vi "Finish.vi"   [LabVIEW 2016]
doc: "This VI is called just before exiting. It is expected to close I/O refnum, save collected data, etc."
uses:
  <vilib>/Rock Robotics/WPI/Utilities/WPI_GetSetVariantRefNum.vi
types:
  T1 = typedef "WPI_MotorControlDeviceRef.ctl" = cluster{"DeviceStatus":errorcluster, "Type":T2, "PWM":cluster{"PWM Channel":T3, "DeadBand":T4}, "CAN":cluster{"Device Number":u8, "SetOutput VI Ref":variant, "GetOutput VI Ref":variant, "Enable VI Ref":variant, "Disable VI Ref":variant, "Data":variant}, "Invert":bool}
  T2 = typedef "WPI_MotorControlType.ctl" = enum16{"PWM", "CAN"}
  T3 = typedef "FPGA_DIOPWMChannel.ctl" = enum8{"PWM 0", "PWM 1", "PWM 2", "PWM 3", "PWM 4", "PWM 5", "PWM 6", "PWM 7", "PWM 8", "PWM 9", "PWM MXP 0", "PWM MXP 1", "PWM MXP 2", "PWM MXP 3", "PWM MXP 4", "PWM MXP 5", "PWM MXP 6", "PWM MXP 7", "PWM MXP 8", "PWM MXP 9", "Invalid"}
  T4 = typedef "WPI_PWMDeadband.ctl" = cluster{"Name":string, "maxPositivePwm":i32, "minPositivePwm":i32, "centerPwm":i32, "maxNegativePwm":i32, "minNegativePwm":i32, "angularRange":u16}
  T5 = typedef "WPI_JoystickDevRef.ctl" = cluster{"Device":T6}
  T6 = typedef "WPI_JoystickDeviceEnum.ctl" = enum16{"USB 0", "USB 1", "USB 2", "USB 3", "USB 4", "USB 5"}
  T7 = typedef "WPI_SolenoidDevRef.ctl" = cluster{"DevStatus":errorcluster, "Pneumatics Control Module":u8, "Forward Solenoid Channel":T8, "Reverse Solenoid Channel":T8}
  T8 = typedef "WPI_SolenoidChannel.ctl" = enum8{"Solenoid 0", "Solenoid 1", "Solenoid 2", "Solenoid 3", "Solenoid 4", "Solenoid 5", "Solenoid 6", "Solenoid 7", "Invalid"}
  T9 = typedef "WPI_GyroDevRef.ctl" = cluster{"DevStatus":errorcluster, "Analog Channel":T10, "Offset":dbl, "Gain (VoltsPerDegree/Second)":dbl, "Gyro Type":enum16{"Analog", "XRS450"}, "Handle":i32, "SPI Bus":T11, "Device Found":bool, "Sample Rate":dbl, "Calibrate On Open":bool}
  T10 = typedef "FPGA_AIChannel.ctl" = enum8{"AI 0", "AI 1", "AI 2", "AI 3", "AI MXP 0", "AI MXP 1", "AI MXP 2", "AI MXP 3", "Invalid"}
  T11 = typedef "spi_bus.ctl" = enum16{"SPI On-Board, CS0", "SPI On-Board, CS1", "SPI On-Board, CS2", "SPI On-Board, CS3", "SPI MXP", "Invalid"}
  T12 = typedef "WPI_EncoderDevRef.ctl" = cluster{"DevStatus":errorcluster, "EncoderIndex":T13, "CounterIndex":T14, "DistancePerCount":dbl, "Decoding Type":T15}
  T13 = typedef "FPGA_EncoderIdx.ctl" = enum8{"Enc 0", "Enc 1", "Enc 2", "Enc 3", "Enc 4", "Enc 5", "Enc 6", "Enc 7", "Invalid"}
  T14 = typedef "FPGA_CounterCtrSystemIndex.ctl" = enum8{"Ctr 0", "Ctr 1", "Ctr 2", "Ctr 3", "Ctr 4", "Ctr 5", "Ctr 6", "Ctr 7", "Invalid"}
  T15 = typedef "WPI_EncoderType.ctl" = enum16{"1x", "2x", "4x"}
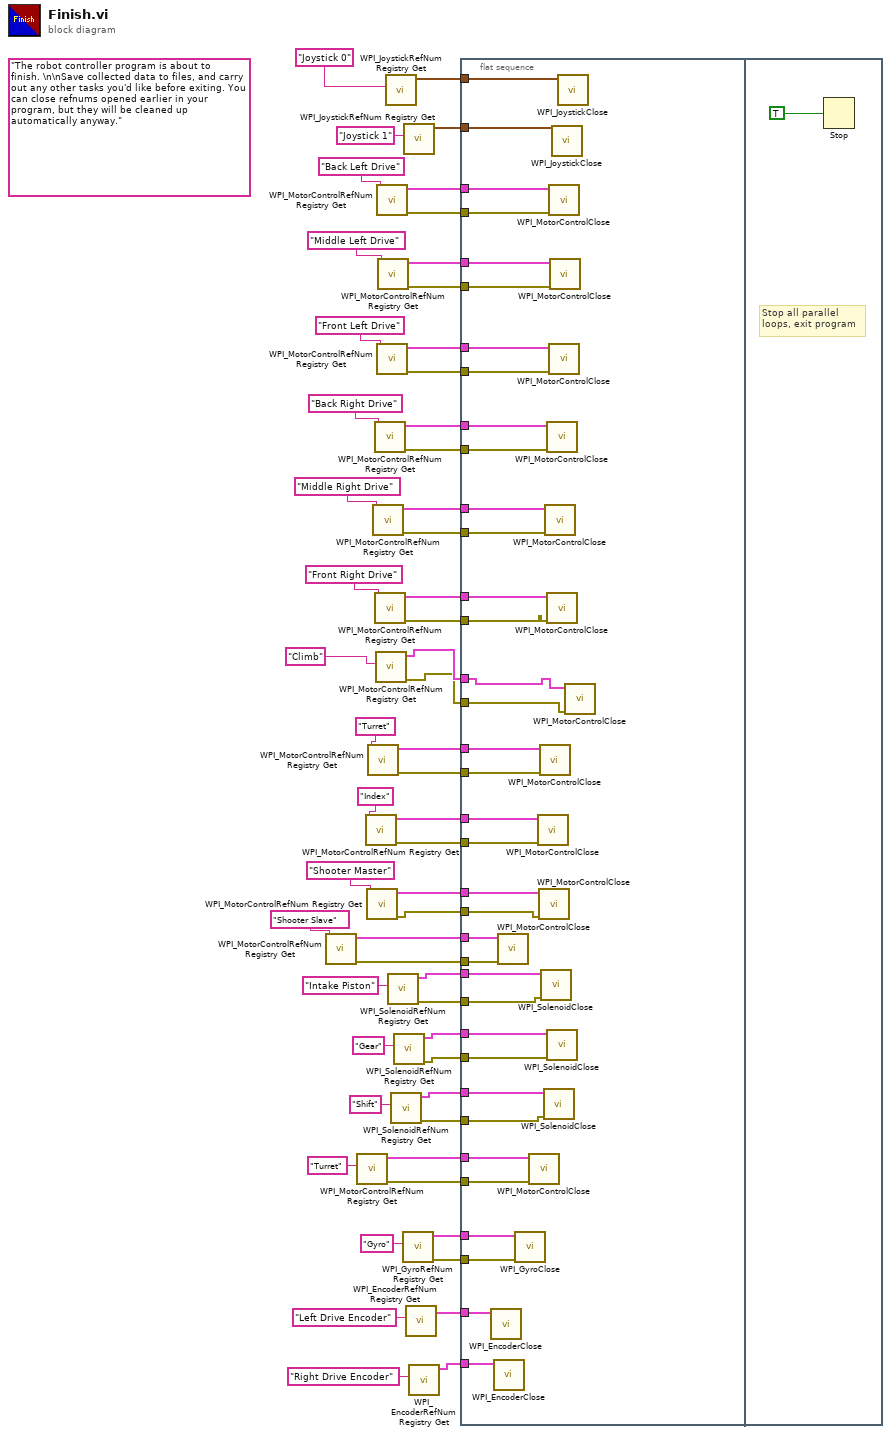
[diagram p0: block diagram]
diagram:
  (unwired) "The robot controller program is about to finish. \n\nSave collected data to files, and carry out any other tasks you'd like before exiting. You can close refnums opened earlier in your program, but they will be cleaned up automatically anyway."
  n1 = call <vilib>:"WPI_MotorControlRefNum Registry Get.vi"("refnum name"="Shooter Slave") -> ("error out"=w21:errorcluster, "MotorControlDevRef"=w31:T1)  [unwired: 9 in]
  n2 = call <vilib>:"WPI_MotorControlRefNum Registry Get.vi"("refnum name"="Turret") -> ("error out"=w16:errorcluster, "MotorControlDevRef"=w28:T1)  [unwired: 9 in]
  n3 = call <vilib>:"WPI_MotorControlRefNum Registry Get.vi"("refnum name"="Index") -> ("error out"=w23:errorcluster, "MotorControlDevRef"=w35:T1)  [unwired: 9 in]
  n4 = call <vilib>:"WPI_MotorControlRefNum Registry Get.vi"("refnum name"="Shooter Master") -> ("error out"=w20:errorcluster, "MotorControlDevRef"=w34:T1)  [unwired: 9 in]
  n5 = call <vilib>:"WPI_MotorControlRefNum Registry Get.vi"("refnum name"="Turret") -> ("error out"=w22:errorcluster, "MotorControlDevRef"=w38:T1)  [unwired: 9 in]
  n6 = call <vilib>:"WPI_MotorControlRefNum Registry Get.vi"("refnum name"="Middle Right Drive") -> ("error out"=w25:errorcluster, "MotorControlDevRef"=w41:T1)  [unwired: 9 in]
  n7 = call <vilib>:"WPI_MotorControlRefNum Registry Get.vi"("refnum name"="Back Right Drive") -> ("error out"=w24:errorcluster, "MotorControlDevRef"=w44:T1)  [unwired: 9 in]
  n8 = call <vilib>:"WPI_MotorControlRefNum Registry Get.vi"("refnum name"="Front Right Drive") -> ("error out"=w26:errorcluster, "MotorControlDevRef"=w40:T1)  [unwired: 9 in]
  n9 = call <vilib>:"WPI_MotorControlRefNum Registry Get.vi"("refnum name"="Climb") -> ("error out"=w10:errorcluster, "MotorControlDevRef"=w11:T1)  [unwired: 9 in]
  n10 = call <vilib>:"WPI_MotorControlRefNum Registry Get.vi"("refnum name"="Back Left Drive") -> ("error out"=w13:errorcluster, "MotorControlDevRef"=w54:T1)  [unwired: 9 in]
  n11 = call <vilib>:"WPI_MotorControlRefNum Registry Get.vi"("refnum name"="Front Left Drive") -> ("error out"=w15:errorcluster, "MotorControlDevRef"=w45:T1)  [unwired: 9 in]
  n12 = call <vilib>:"WPI_MotorControlRefNum Registry Get.vi"("refnum name"="Middle Left Drive") -> ("error out"=w14:errorcluster, "MotorControlDevRef"=w48:T1)  [unwired: 9 in]
  n13 = call <vilib>:"WPI_JoystickRefNum Registry Get.vi"("refnum name"="Joystick 0") -> ("JoystickDevRef"=w53:T5)  [unwired: 1 in, 9 out]
  n14 = call <vilib>:"WPI_SolenoidRefNum Registry Get.vi"("refnum name"="Intake Piston") -> ("error out"=w19:errorcluster, "SolenoidDevRef"=w51:T7)  [unwired: 9 in]
  n15 = call <vilib>:"WPI_SolenoidRefNum Registry Get.vi"("refnum name"="Shift") -> ("error out"=w17:errorcluster, "SolenoidDevRef"=w29:T7)  [unwired: 9 in]
  n16 = call <vilib>:"WPI_SolenoidRefNum Registry Get.vi"("refnum name"="Gear") -> ("error out"=w18:errorcluster, "SolenoidDevRef"=w50:T7)  [unwired: 9 in]
  n17 = call <vilib>:"WPI_GyroRefNum Registry Get.vi"("refnum name"="Gyro") -> ("error out"=w6:errorcluster, "GyroDevRef"=w7:T9)  [unwired: 9 in]
  n18 = call <vilib>:"WPI_JoystickRefNum Registry Get.vi"("refnum name"="Joystick 1") -> ("JoystickDevRef"=w8:T5)  [unwired: 9 in, 1 out]
  n19 = call <vilib>:"WPI_EncoderRefNum Registry Get.vi"("refnum name"="Left Drive Encoder") -> ("EncoderDevRef"=w2:T12)  [unwired: 9 in, 1 out]
  n20 = call <vilib>:"WPI_EncoderRefNum Registry Get.vi"("refnum name"="Right Drive Encoder") -> ("EncoderDevRef"=w1:T12)  [unwired: 9 in, 1 out]
  n21 = flat-sequence {
    tunnel: w54 -> [w89]
    tunnel: w53 -> [w92]
    tunnel: w51 -> [w91]
    tunnel: w50 -> [w90]
    tunnel: w48 -> [w88]
    tunnel: w45 -> [w87]
    tunnel: w44 -> [w86]
    tunnel: w41 -> [w85]
    tunnel: w40 -> [w84]
    tunnel: w11 -> [w63]
    tunnel: w38 -> [w83]
    tunnel: w35 -> [w82]
    tunnel: w34 -> [w81]
    tunnel: w31 -> [w80]
    tunnel: w29 -> [w79]
    tunnel: w28 -> [w78]
    tunnel: w10 -> [w62]
    tunnel: w26 -> [w77]
    tunnel: w25 -> [w76]
    tunnel: w24 -> [w75]
    tunnel: w23 -> [w74]
    tunnel: w22 -> [w73]
    tunnel: w21 -> [w72]
    tunnel: w20 -> [w71]
    tunnel: w19 -> [w70]
    tunnel: w18 -> [w69]
    tunnel: w17 -> [w68]
    tunnel: w16 -> [w67]
    tunnel: w15 -> [w66]
    tunnel: w14 -> [w65]
    tunnel: w13 -> [w64]
    tunnel: w8 -> [w61]
    tunnel: w7 -> [w60]
    tunnel: w6 -> [w59]
    tunnel: w2 -> [w58]
    tunnel: w1 -> [w57]
    frame #0 {
      n22 = call <vilib>:"WPI_EncoderClose.vi"("EncoderDevRef"=w58) -> ()  [unwired: 10 in, 1 out]
      n23 = call <vilib>:"WPI_EncoderClose.vi"("EncoderDevRef"=w57) -> ()  [unwired: 10 in, 1 out]
      n24 = call <vilib>:"WPI_MotorControlClose.vi"("error in"=w72, "MotorControlDevRef"=w80) -> ()  [unwired: 9 in, 1 out]
      n25 = call <vilib>:"WPI_GyroClose.vi"("error in"=w59, "GyroDevRef"=w60) -> ()  [unwired: 9 in, 1 out]
      n26 = call <vilib>:"WPI_MotorControlClose.vi"("error in"=w67, "MotorControlDevRef"=w78) -> ()  [unwired: 9 in, 1 out]
      n27 = call <vilib>:"WPI_MotorControlClose.vi"("error in"=w74, "MotorControlDevRef"=w82) -> ()  [unwired: 9 in, 1 out]
      n28 = call <vilib>:"WPI_MotorControlClose.vi"("error in"=w71, "MotorControlDevRef"=w81) -> ()  [unwired: 9 in, 1 out]
      n29 = call <vilib>:"WPI_MotorControlClose.vi"("error in"=w73, "MotorControlDevRef"=w83) -> ()  [unwired: 9 in, 1 out]
      n30 = call <vilib>:"WPI_SolenoidClose.vi"("error in (no error)"=w70, "SolenoidDevRef"=w91) -> ()  [unwired: 9 in, 1 out]
      n31 = call <vilib>:"WPI_SolenoidClose.vi"("error in (no error)"=w68, "SolenoidDevRef"=w79) -> ()  [unwired: 9 in, 1 out]
      n32 = call <vilib>:"WPI_MotorControlClose.vi"("error in"=w76, "MotorControlDevRef"=w85) -> ()  [unwired: 9 in, 1 out]
      n33 = call <vilib>:"WPI_MotorControlClose.vi"("error in"=w75, "MotorControlDevRef"=w86) -> ()  [unwired: 9 in, 1 out]
      n34 = call <vilib>:"WPI_MotorControlClose.vi"("error in"=w77, "MotorControlDevRef"=w84) -> ()  [unwired: 9 in, 1 out]
      n35 = call <vilib>:"WPI_SolenoidClose.vi"("error in (no error)"=w69, "SolenoidDevRef"=w90) -> ()  [unwired: 9 in, 1 out]
      n36 = call <vilib>:"WPI_MotorControlClose.vi"("error in"=w64, "MotorControlDevRef"=w89) -> ()  [unwired: 9 in, 1 out]
      n37 = call <vilib>:"WPI_MotorControlClose.vi"("error in"=w66, "MotorControlDevRef"=w87) -> ()  [unwired: 9 in, 1 out]
      n38 = call <vilib>:"WPI_MotorControlClose.vi"("error in"=w65, "MotorControlDevRef"=w88) -> ()  [unwired: 9 in, 1 out]
      n39 = call <vilib>:"WPI_JoystickClose.vi"("JoystickDevRef"=w61) -> ()  [unwired: 11 out]
      n40 = call <vilib>:"WPI_JoystickClose.vi"("JoystickDevRef"=w92) -> ()  [unwired: 11 out]
      n41 = call <vilib>:"WPI_MotorControlClose.vi"("error in"=w62, "MotorControlDevRef"=w63) -> ()  [unwired: 9 in, 1 out]
    }
    frame #1 {
      # "Stop all parallel\nloops, exit program"
      n42 = Stop(stop? (T)=TRUE ("Quit")) -> ()
    }
  }
